vi "Visible_Ch_Init _11-20.vi"   [LabVIEW 2017]
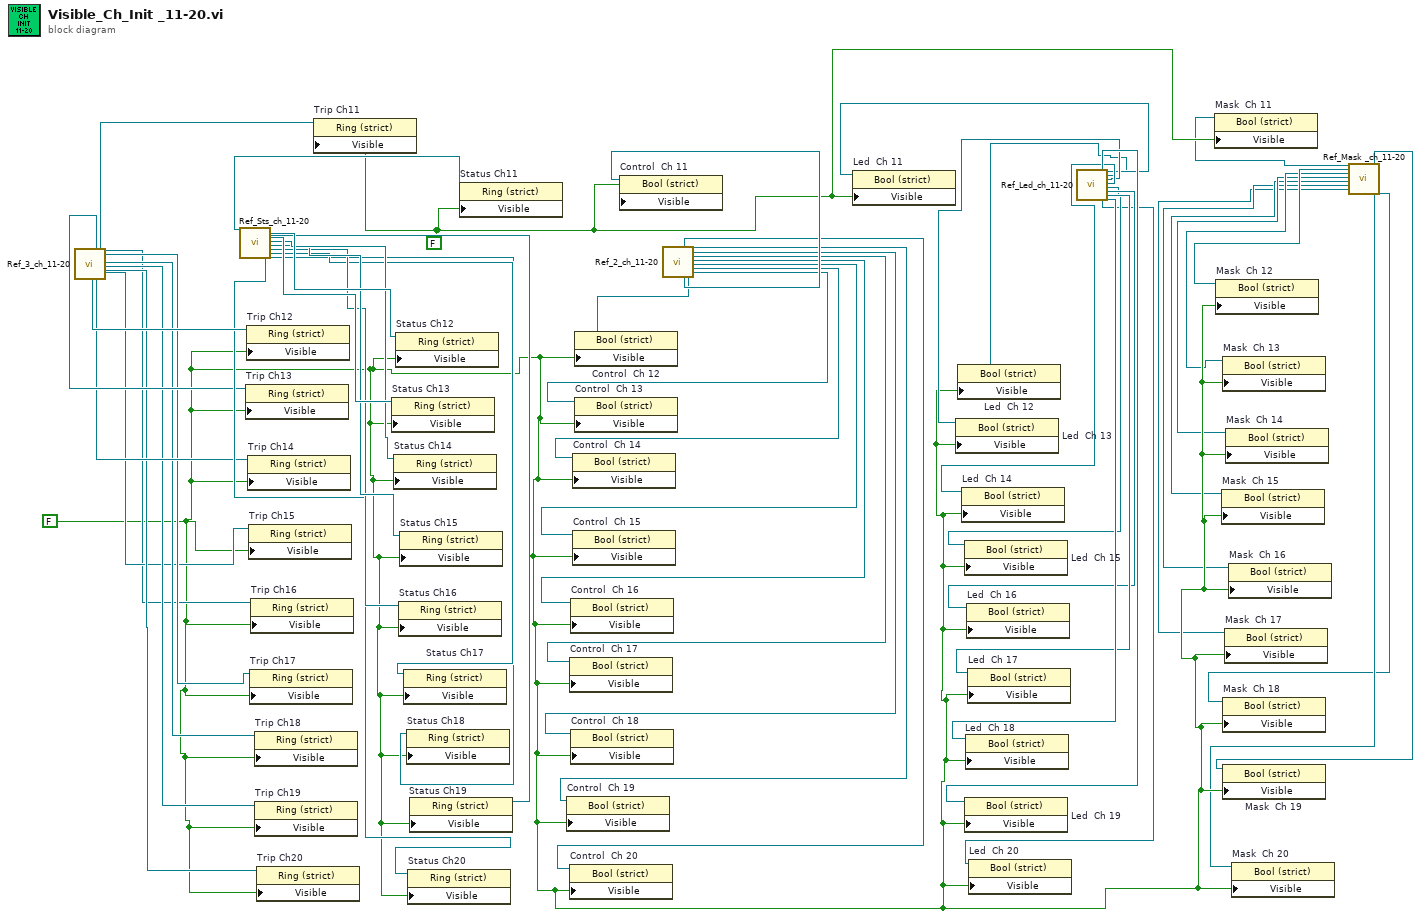
[diagram p0: block diagram]
diagram:
  w11 = FALSE
  w12 = FALSE
  n1 = call "Ref_3_ch_11-20.vi"() -> ("Trip  Ch 11 out"=w52:refnum<vi>, "Trip  Ch 12 out"=w49:refnum<vi>, "Trip  Ch 13 out"=w33:refnum<vi>, "Trip  Ch 14 out"=w32:refnum<vi>, "Trip  Ch 15 out"=w14:refnum<vi>, "Trip  Ch 16 out"=w13:refnum<vi>, "Trip  Ch 17 out"=w31:refnum<vi>, "Trip  Ch 18 out"=w30:refnum<vi>, "Trip  Ch 19 out"=w29:refnum<vi>, "Trip  Ch 20 out"=w28:refnum<vi>)  [unwired: 18 in]
  n2 = call "Ref_Sts_ch_11-20.vi"() -> ("Status Ch 19 out"=w35:refnum<vi>, "Status Ch 20 out"=w34:refnum<vi>, "Status Ch 11 out"=w51:refnum<vi>, "Status Ch 12 out"=w41:refnum<vi>, "Status Ch 13 out"=w40:refnum<vi>, "Status Ch 14 out"=w39:refnum<vi>, "Status Ch 15 out"=w38:refnum<vi>, "Status Ch 16 out"=w37:refnum<vi>, "Status Ch 17 out"=w36:refnum<vi>, "Status Ch 18 out"=w25:refnum<vi>)  [unwired: 18 in]
  n3 = property on="Trip Ch13" class="Ring (strict)"(reference=w33, "Visible"=w11) -> ()  [unwired: 1 in, 2 out]
  n4 = property on="Trip Ch12" class="Ring (strict)"(reference=w49, "Visible"=w11) -> ()  [unwired: 1 in, 2 out]
  n5 = property on="Trip Ch14" class="Ring (strict)"(reference=w32, "Visible"=w11) -> ()  [unwired: 1 in, 2 out]
  n6 = property on="Trip Ch15" class="Ring (strict)"(reference=w14, "Visible"=w11) -> ()  [unwired: 1 in, 2 out]
  n7 = property on="Trip Ch17" class="Ring (strict)"(reference=w31, "Visible"=w11) -> ()  [unwired: 1 in, 2 out]
  n8 = property on="Trip Ch16" class="Ring (strict)"(reference=w13, "Visible"=w11) -> ()  [unwired: 1 in, 2 out]
  n9 = property on="Trip Ch18" class="Ring (strict)"(reference=w30, "Visible"=w11) -> ()  [unwired: 1 in, 2 out]
  n10 = property on="Trip Ch19" class="Ring (strict)"(reference=w29, "Visible"=w11) -> ()  [unwired: 1 in, 2 out]
  n11 = property on="Trip Ch20" class="Ring (strict)"(reference=w28, "Visible"=w11) -> ()  [unwired: 1 in, 2 out]
  n12 = property on="Trip Ch11" class="Ring (strict)"(reference=w52, "Visible"=w12) -> ()  [unwired: 1 in, 2 out]
  n13 = property on="Status Ch13" class="Ring (strict)"(reference=w40, "Visible"=w11) -> ()  [unwired: 1 in, 2 out]
  n14 = property on="Status Ch14" class="Ring (strict)"(reference=w39, "Visible"=w11) -> ()  [unwired: 1 in, 2 out]
  n15 = property on="Status Ch12" class="Ring (strict)"(reference=w41, "Visible"=w11) -> ()  [unwired: 1 in, 2 out]
  n16 = property on="Status Ch16" class="Ring (strict)"(reference=w37, "Visible"=w11) -> ()  [unwired: 1 in, 2 out]
  n17 = property on="Status Ch15" class="Ring (strict)"(reference=w38, "Visible"=w11) -> ()  [unwired: 1 in, 2 out]
  n18 = property on="Status Ch17" class="Ring (strict)"(reference=w36, "Visible"=w11) -> ()  [unwired: 1 in, 2 out]
  n19 = property on="Status Ch18" class="Ring (strict)"(reference=w25, "Visible"=w11) -> ()  [unwired: 1 in, 2 out]
  n20 = property on="Status Ch20" class="Ring (strict)"(reference=w34, "Visible"=w11) -> ()  [unwired: 1 in, 2 out]
  n21 = property on="Status Ch19" class="Ring (strict)"(reference=w35, "Visible"=w11) -> ()  [unwired: 1 in, 2 out]
  n22 = property on="Status Ch11" class="Ring (strict)"(reference=w51, "Visible"=w12) -> ()  [unwired: 1 in, 2 out]
  n23 = call "Ref_2_ch_11-20.vi"() -> ("Control  Ch 20 out"=w42:refnum<vi>, "Control  Ch 11 out"=w50:refnum<vi>, "Control  Ch 19 out"=w43:refnum<vi>, "Control  Ch 12 out"=w48:refnum<vi>, "Control  Ch 18 out"=w44:refnum<vi>, "Control  Ch 17 out"=w45:refnum<vi>, "Control  Ch 16 out"=w26:refnum<vi>, "Control  Ch 15 out"=w46:refnum<vi>, "Control  Ch 14 out"=w47:refnum<vi>, "Control  Ch 13 out"=w27:refnum<vi>)  [unwired: 17 in, 1 out]
  n24 = property on="Control  Ch 19" class="Bool (strict)"(reference=w43, "Visible"=w11) -> ()  [unwired: 1 in, 2 out]
  n25 = property on="Control  Ch 17" class="Bool (strict)"(reference=w45, "Visible"=w11) -> ()  [unwired: 1 in, 2 out]
  n26 = property on="Control  Ch 20" class="Bool (strict)"(reference=w42, "Visible"=w11) -> ()  [unwired: 1 in, 2 out]
  n27 = property on="Control  Ch 16" class="Bool (strict)"(reference=w26, "Visible"=w11) -> ()  [unwired: 1 in, 2 out]
  n28 = property on="Control  Ch 18" class="Bool (strict)"(reference=w44, "Visible"=w11) -> ()  [unwired: 1 in, 2 out]
  n29 = property on="Control  Ch 14" class="Bool (strict)"(reference=w47, "Visible"=w11) -> ()  [unwired: 1 in, 2 out]
  n30 = property on="Control  Ch 15" class="Bool (strict)"(reference=w46, "Visible"=w11) -> ()  [unwired: 1 in, 2 out]
  n31 = property on="Control  Ch 12" class="Bool (strict)"(reference=w48, "Visible"=w11) -> ()  [unwired: 1 in, 2 out]
  n32 = property on="Control  Ch 13" class="Bool (strict)"(reference=w27, "Visible"=w11) -> ()  [unwired: 1 in, 2 out]
  n33 = property on="Control  Ch 11" class="Bool (strict)"(reference=w50, "Visible"=w12) -> ()  [unwired: 1 in, 2 out]
  n34 = call "Ref_Led_ch_11-20.vi"() -> ("Led Ch 19 out"=w24:refnum<vi>, "Led Ch 20 out"=w17:refnum<vi>, "Led Ch 11 out"=w16:refnum<vi>, "Led Ch 12 out"=w15:refnum<vi>, "Led Ch 13 out"=w18:refnum<vi>, "Led Ch 14 out"=w19:refnum<vi>, "Led Ch 15 out"=w20:refnum<vi>, "Led Ch 16 out"=w21:refnum<vi>, "Led Ch 17 out"=w22:refnum<vi>, "Led Ch 18 out"=w23:refnum<vi>)  [unwired: 18 in]
  n35 = property on="Led  Ch 11" class="Bool (strict)"(reference=w16, "Visible"=w12) -> ()  [unwired: 1 in, 2 out]
  n36 = property on="Led  Ch 13" class="Bool (strict)"(reference=w18, "Visible"=w11) -> ()  [unwired: 1 in, 2 out]
  n37 = property on="Led  Ch 12" class="Bool (strict)"(reference=w15, "Visible"=w11) -> ()  [unwired: 1 in, 2 out]
  n38 = property on="Led  Ch 14" class="Bool (strict)"(reference=w19, "Visible"=w11) -> ()  [unwired: 1 in, 2 out]
  n39 = property on="Led  Ch 15" class="Bool (strict)"(reference=w20, "Visible"=w11) -> ()  [unwired: 1 in, 2 out]
  n40 = property on="Led  Ch 19" class="Bool (strict)"(reference=w24, "Visible"=w11) -> ()  [unwired: 1 in, 2 out]
  n41 = property on="Led  Ch 18" class="Bool (strict)"(reference=w23, "Visible"=w11) -> ()  [unwired: 1 in, 2 out]
  n42 = property on="Led  Ch 16" class="Bool (strict)"(reference=w21, "Visible"=w11) -> ()  [unwired: 1 in, 2 out]
  n43 = property on="Led  Ch 17" class="Bool (strict)"(reference=w22, "Visible"=w11) -> ()  [unwired: 1 in, 2 out]
  n44 = property on="Led  Ch 20" class="Bool (strict)"(reference=w17, "Visible"=w11) -> ()  [unwired: 1 in, 2 out]
  n45 = call "Ref_Mask _ch_11-20.vi"() -> ("Mask Ch 19 out"=w1:refnum<vi>, "Mask Ch 20 out"=w3:refnum<vi>, "Mask Ch 11 out"=w10:refnum<vi>, "Mask Ch 12 out"=w9:refnum<vi>, "Mask Ch 13 out"=w8:refnum<vi>, "Mask Ch 14 out"=w7:refnum<vi>, "Mask Ch 15 out"=w6:refnum<vi>, "Mask Ch 16 out"=w5:refnum<vi>, "Mask Ch 17 out"=w4:refnum<vi>, "Mask Ch 18 out"=w2:refnum<vi>)  [unwired: 18 in]
  n46 = property on="Mask  Ch 11" class="Bool (strict)"(reference=w10, "Visible"=w12) -> ()  [unwired: 1 in, 2 out]
  n47 = property on="Mask  Ch 12" class="Bool (strict)"(reference=w9, "Visible"=w11) -> ()  [unwired: 1 in, 2 out]
  n48 = property on="Mask  Ch 15" class="Bool (strict)"(reference=w6, "Visible"=w11) -> ()  [unwired: 1 in, 2 out]
  n49 = property on="Mask  Ch 13" class="Bool (strict)"(reference=w8, "Visible"=w11) -> ()  [unwired: 1 in, 2 out]
  n50 = property on="Mask  Ch 18" class="Bool (strict)"(reference=w2, "Visible"=w11) -> ()  [unwired: 1 in, 2 out]
  n51 = property on="Mask  Ch 19" class="Bool (strict)"(reference=w1, "Visible"=w11) -> ()  [unwired: 1 in, 2 out]
  n52 = property on="Mask  Ch 17" class="Bool (strict)"(reference=w4, "Visible"=w11) -> ()  [unwired: 1 in, 2 out]
  n53 = property on="Mask  Ch 14" class="Bool (strict)"(reference=w7, "Visible"=w11) -> ()  [unwired: 1 in, 2 out]
  n54 = property on="Mask  Ch 16" class="Bool (strict)"(reference=w5, "Visible"=w11) -> ()  [unwired: 1 in, 2 out]
  n55 = property on="Mask  Ch 20" class="Bool (strict)"(reference=w3, "Visible"=w11) -> ()  [unwired: 1 in, 2 out]
